vi "rs3_ExtractColor3.vi"(0 "White Balance":bool, 1 "24bit Color Array":u8[](array[numeric]), 3 "Alpha":dbl, 5 "Red":dbl=2.0, 7 "Color format":enum16{"Monochrome", "RGB internal (RGB)"}(ring), 9 "Green":dbl=1.0, 10 "Depth Y":i32=360, 11 "Blue":dbl=2.0, 12 "RGB  X":i32=640, 14 "RGB Y":i32=480, 15 "Depth X":i32=480) -> (4 "Norm Mesh Color":T1(array[cluster]))   [LabVIEW 2017, in "libRealSense3.lvlib"]
doc: "Extract the color in a format required for plotting a pointcloud into 3D picture indication"
uses:
  libRealSense3.lvlib
panel:
  out "Ratio X":dbl=1.3333333333333333
  out "Ratio Y":dbl=1.3333333333333333
  # "RS3 Extract Color for PointCloud"
  # "(C) Intel Corp. 2017,  AGJ"
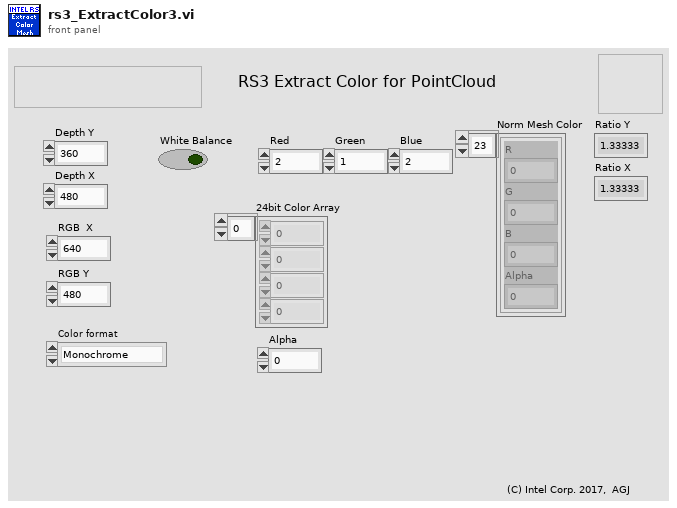
[diagram p1: front panel]
types:
  T1 = cluster{"R":dbl, "G":dbl, "B":dbl, "Alpha":dbl}[]
  T2 = cluster{"upper limit":dbl, "upper limit":dbl, "upper limit":dbl, "Alpha":dbl}[]
  T3 = cluster{"upper limit":dbl, "upper limit":dbl, "upper limit":dbl, u8}
  T4 = cluster{"upper limit":dbl, "upper limit":dbl, "upper limit":dbl, "Alpha":dbl}
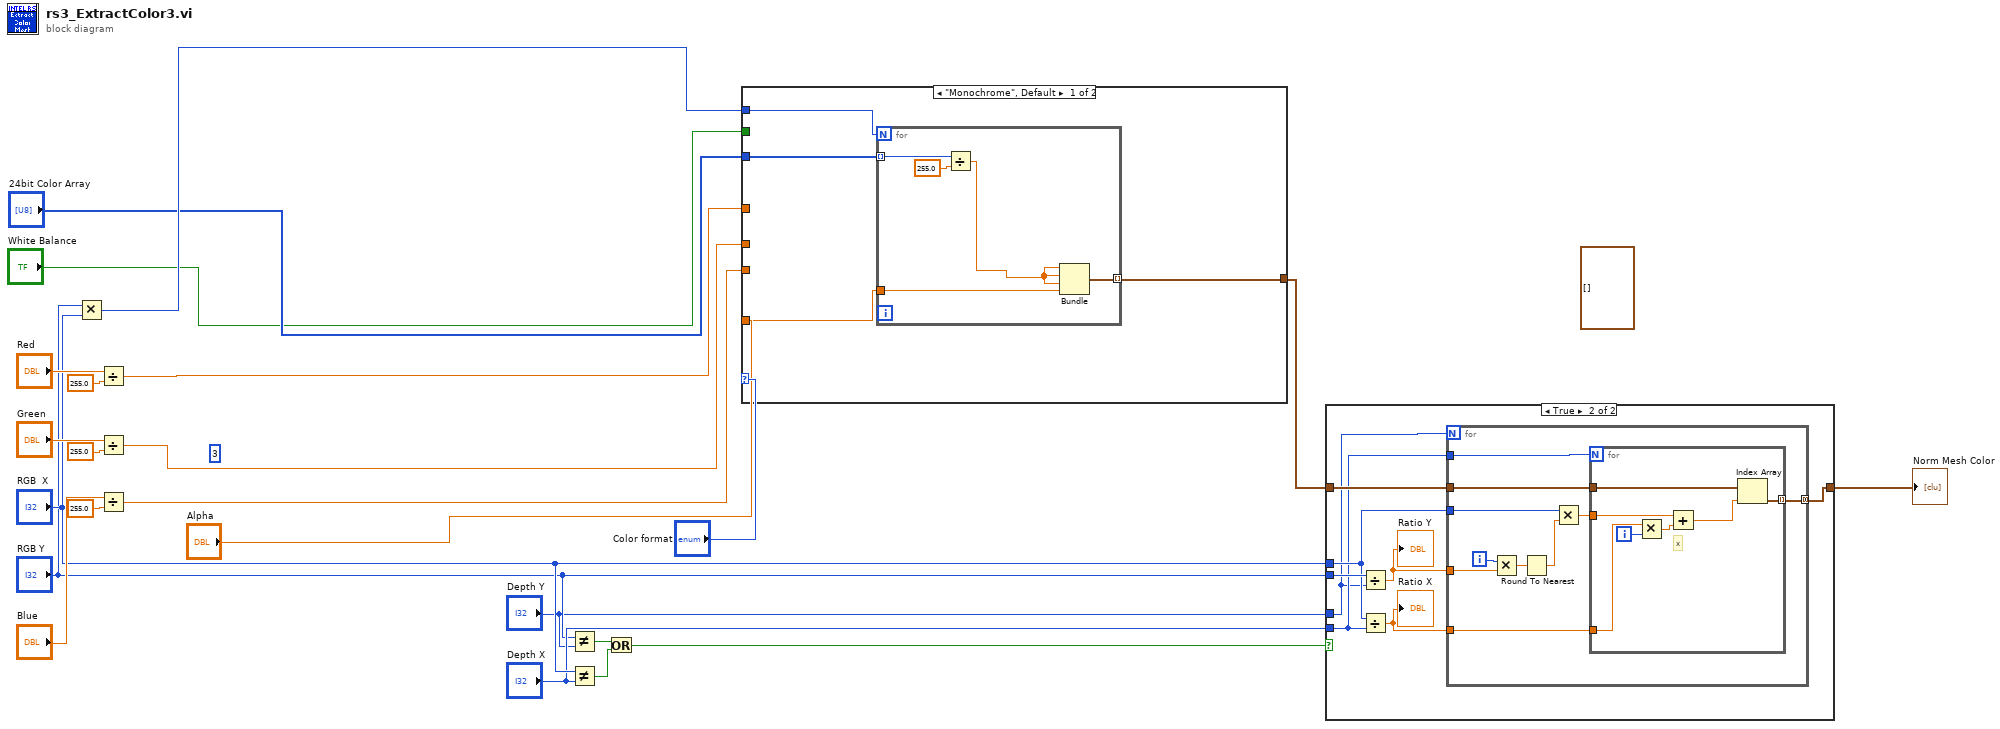
[diagram p0: block diagram]
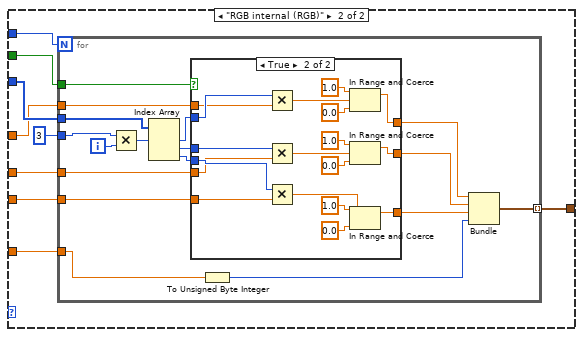
[diagram p2: hidden frame]
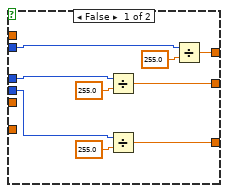
[diagram p3: hidden frame]
diagram:
  (unwired) T2 []
  (unwired) 3 ("# of bytes/number")
  n1 = Multiply(x="RGB Y", y="RGB  X") -> (x*y=w9:i32)
  n2 = Divide(x="Red", y=255.0 ("upper limit")) -> (x/y=w7:dbl)
  n3 = Divide(x="Green", y=255.0 ("upper limit")) -> (x/y=w6:dbl)
  n4 = Divide(x="Blue", y=255.0 ("upper limit")) -> (x/y=w2:dbl)
  n5 = Not Equal?(x="RGB Y", y="Depth Y") -> (x != y?=w12:bool)
  n6 = Not Equal?(x="RGB  X", y="Depth X") -> (x != y?=w15:bool)
  n7 = Or(x=w12, y=w15) -> (x .or. y?=w11:bool)
  n8 = case shown="\"Monochrome\", Default" "Color format" {
    tunnel: "24bit Color Array" -> [w26 w41]
    tunnel: w7 -> [_ w39]
    tunnel: w2 -> [_ w38]
    tunnel: w6 -> [_ w37]
    tunnel: "Alpha" -> [w25 w36]
    tunnel: w9 -> [w27 w35]
    tunnel: [w24 w34] -> w1
    tunnel: "White Balance" -> [_ w33]
    frame "Monochrome", Default {
      n9 = for {
        N: w27 -> [_]
        tunnel: w26 -> [w30] mode=indexing
        tunnel: [w32] -> w24 mode=indexing
        tunnel: w25 -> [w29]
        n10 = Divide(x=w30, y=255.0 ("upper limit")) -> (x/y=w28:dbl)
        n11 = Bundle(w28, w28, w28, "Alpha"=w29) -> (w32:cluster{dbl, dbl, dbl, "Alpha":dbl})  [unwired: 1 in]
      }
    }
    frame "RGB internal (RGB)" {
      n12 = for {
        N: w35 -> [_]
        tunnel: w41 -> [w56]
        tunnel: 3 ("# of bytes/number") -> [w55]
        tunnel: [w54] -> w34 mode=indexing
        tunnel: w39 -> [w50]
        tunnel: w37 -> [w49]
        tunnel: w38 -> [w48]
        tunnel: w36 -> [w46]
        tunnel: w33 -> [w47]
        i -> [w58]
        n13 = Multiply(x=w55, y=w58) -> (x*y=w57:i32)
        n14 = Index Array(array=w56, index #1=w57) -> (element #1=w53:u8, element #2=w52:u8, element #3=w51:u8)  [unwired: 2 in]
        n15 = case shown="True" w47 {
          tunnel: w53 -> [w66 w85]
          tunnel: w52 -> [w62 w84]
          tunnel: w51 -> [w61 w83]
          tunnel: w50 -> [_ w82]
          tunnel: w49 -> [_ w81]
          tunnel: w48 -> [_ w80]
          tunnel: [w65 w70] -> w42
          tunnel: [w59 w69] -> w43
          tunnel: [w60 w68] -> w44
          frame False {
            n16 = Divide(x=w62, y=255.0 ("upper limit")) -> (x/y=w59:dbl)
            n17 = Divide(x=w61, y=255.0 ("upper limit")) -> (x/y=w60:dbl)
            n18 = Divide(x=w66, y=255.0 ("upper limit")) -> (x/y=w65:dbl)
          }
          frame True {
            n19 = Multiply(x=w85, y=w82) -> (x*y=w79:dbl)
            n20 = Multiply(x=w84, y=w81) -> (x*y=w73:dbl)
            n21 = Multiply(x=w83, y=w80) -> (x*y=w74:dbl)
            n22 = In Range and Coerce(upper limit=1.0, x=w79, lower limit=0.0) -> (coerced(x)=w70:dbl)  [unwired: 1 out]
            n23 = In Range and Coerce(upper limit=1.0, x=w73, lower limit=0.0) -> (coerced(x)=w69:dbl)  [unwired: 1 out]
            n24 = In Range and Coerce(upper limit=1.0, x=w74, lower limit=0.0) -> (coerced(x)=w68:dbl)  [unwired: 1 out]
          }
        }
        n25 = To Unsigned Byte Integer(number=w46) -> (unsigned 8bit integer=w45:u8)
        n26 = Bundle("upper limit"=w42, "upper limit"=w43, "upper limit"=w44, w45) -> (w54:T3)  [unwired: 1 in]
      }
    }
  }
  n27 = case shown="True" w11 {
    tunnel: w1 -> [w86 w94]
    tunnel: [w86 w93] -> w10
    tunnel: "RGB Y" -> [_ w92]
    tunnel: "RGB  X" -> [_ w91]
    tunnel: "Depth X" -> [_ w90]
    tunnel: "Depth Y" -> [_ w89]
    frame False {
    }
    frame True {
      n28 = Divide(x=w92, y=w89) -> (x/y=w87:dbl)
      "Ratio Y" <- w87
      n29 = Divide(x=w91, y=w90) -> (x/y=w88:dbl)
      "Ratio X" <- w88
      n30 = for {
        N: w89 -> [_]
        tunnel: w90 -> [w104]
        tunnel: w88 -> [w103]
        tunnel: w87 -> [w100]
        tunnel: w91 -> [w96]
        tunnel: w94 -> [w102]
        tunnel: [w101] -> w93 mode=concatenating
        i -> [w98]
        n31 = Multiply(x=w98, y=w100) -> (x*y=w99:dbl)
        n32 = Round To Nearest(number=w99) -> (nearest integer value=w97:dbl)
        n33 = Multiply(x=w96, y=w97) -> (x*y=w95:dbl)
        n34 = for {
          N: w104 -> [_]
          tunnel: w103 -> [w110]
          tunnel: w102 -> [w108]
          tunnel: [w107] -> w101 mode=indexing
          tunnel: w95 -> [w106]
          i -> [w111]
          # "x"
          n35 = Multiply(x=w110, y=w111) -> (x*y=w109:dbl)
          n36 = Add(x=w106, y=w109) -> (x+y=w105:dbl)
          n37 = Index Array(array=w108, index=w105) -> (element=w107:T4)
        }
      }
    }
  }
  "Norm Mesh Color" <- w10
